vi "noise range test tool.vi"() -> ()   [LabVIEW 2014]
panel:
  out "Waveform Chart":dbl(graph)
  in  "Stop Button":bool
  in  "noise amplitude":u16=32768 caption="amplitude"
  in  "noise reduction factor":i16
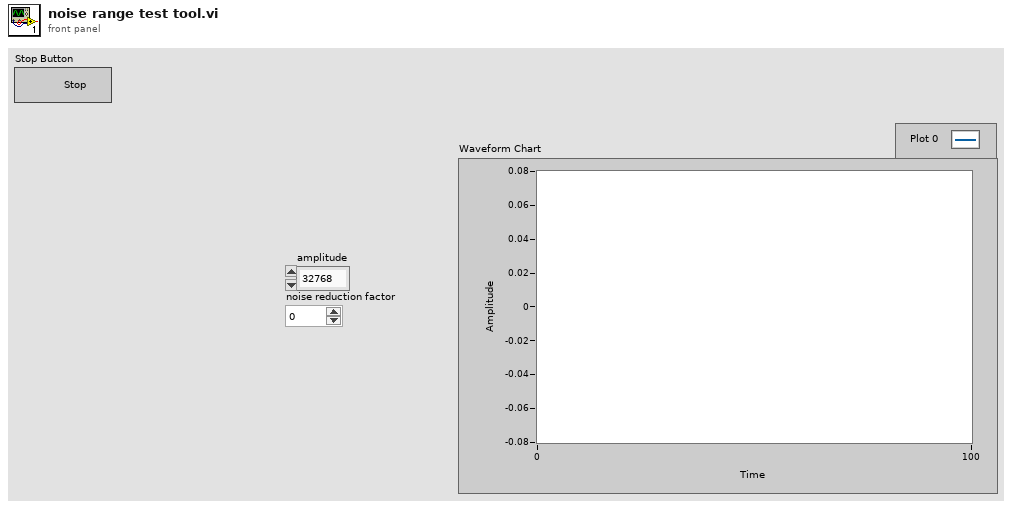
[diagram p1: front panel]
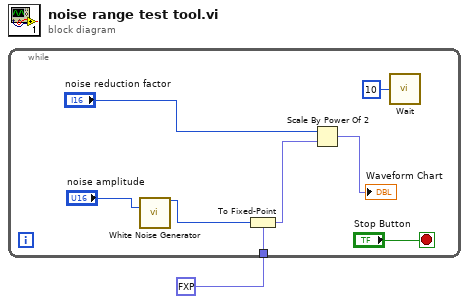
[diagram p0: block diagram]
diagram:
  n1 = while {
    tunnel: fxp<+/-,43,21> 0.0 ("x*y") -> [w4]
    stop <- "Stop Button" stop-if-true
    n2 = call "White Noise Generator"("amplitude"="noise amplitude") -> ("white noise out"=w3:i16)  [unwired: 14 in]
    n3 = To Fixed-Point(fixed-point type=w4, number=w3) -> (fixed-point=w2:fxp<+/-,43,21>)
    n4 = Scale By Power Of 2(n="noise reduction factor", x=w2) -> (x*2^n=→"Waveform Chart":fxp<+/-,43,21>)
    n5 = call "Wait"("Count(mSec)"=u32 10) -> ()  [unwired: 1 out]
  }
